vi "Disable All Axes.vi"(8 "error in (no error)":errorcluster, 11 "Gantry in":refnum<class "A3200.lvclass">) -> (0 "error out":errorcluster, 3 "Gantry out":refnum<class "A3200.lvclass">)   [LabVIEW 2020, in "A3200.lvclass"]
uses:
  A3200.lvclass
  A3200.lvclass/A3200.ctl
  Drivers/Aerotech A3200/Aerotech.lvlib
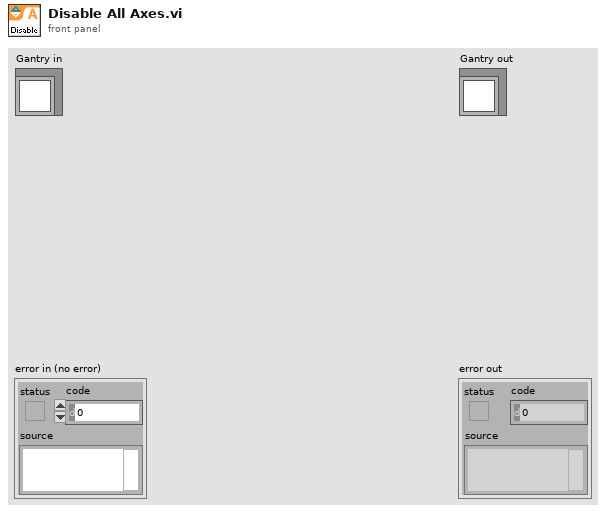
[diagram p1: front panel]
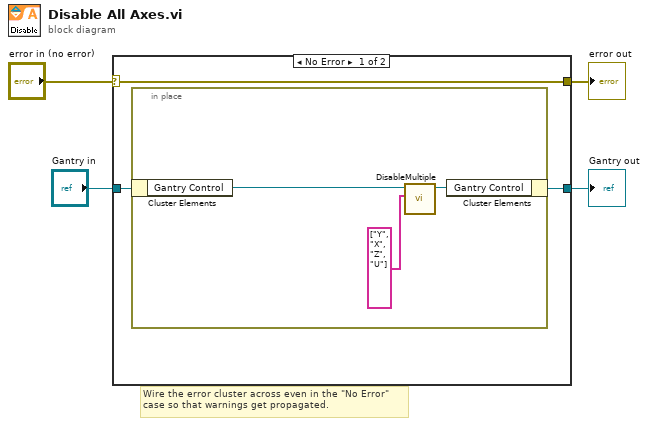
[diagram p0: block diagram]
diagram:
  # "Wire the error cluster across even in the \"No Error\"\ncase so that warnings get propagated."
  n1 = case shown="No Error" "error in (no error)" {
    selector: "error in (no error)" -> [w7 w12]
    tunnel: [w7 w12] -> w3
    tunnel: [w5 w11] -> w1
    tunnel: "Gantry in" -> [w6 w11]
    frame No Error {
      n2 = in-place {
        n3 = in-place-cluster #1(w6) -> ("Gantry Control"=w8:refnum<k24>)
        n4 = call "DisableMultiple.vi"("axis names"=string[] ["Y", "X", "Z", "U"], "controller in"=w8) -> ("controller out"=w10:refnum<k24>)  [unwired: 8 in, 1 out]
        n5 = in-place-cluster #1("Gantry Control"=w10) -> (w5:refnum<class "A3200.lvclass">)
      }
    }
    frame Error {
    }
  }
  "error out" <- w3
  "Gantry out" <- w1
